vi "CallChainSearch.vi"(10 "Root VI name":string, 11 "CallChain":string[](array[string])) -> (2 "Found index":i32, 3 "Clone ID":string)   [LabVIEW 2019]
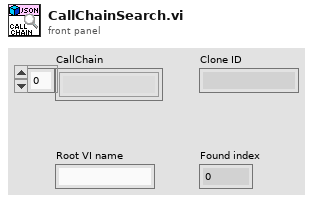
[diagram p1: front panel]
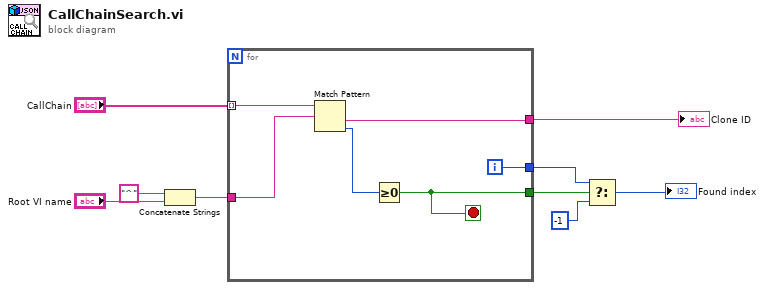
[diagram p0: block diagram]
diagram:
  n1 = Concatenate Strings("^" ("string"), "Root VI name") -> (w8:string)
  n2 = for {
    tunnel: "CallChain" -> [w15] mode=indexing
    tunnel: w8 -> [w14]
    tunnel: [w12] -> w1
    tunnel: [w11] -> w5
    tunnel: [w10] -> w4
    i -> [w10]
    stop <- w11 stop-if-true
    n3 = Match Pattern(string=w15, regular expression=w14) -> (after substring=w12:string, offset past match=w13:i32)  [unwired: 1 in, 2 out]
    n4 = Greater Or Equal To 0?(x=w13) -> (x >= 0?=w11:bool)
  }
  "Clone ID" <- w1
  n5 = Select(t=w4, s=w5, f=-1) -> (s? t:f=→"Found index":i32)
